vi "toStringArray.vi"(8 "error in (no error)":errorcluster, 11 "SingleTone in":refnum<class "SingleTone.lvclass">) -> (0 "error out":errorcluster, 2 "eventStringArray":string[](array[string]), 3 "SingleTone out":refnum<class "SingleTone.lvclass">)   [LabVIEW 2011, in "Tools.lvlib" / "Scripting.lvlib" / "SingleTone.lvclass"]
uses:
  SingleTone.lvclass
  ScriptEvent.lvclass
  SingleTone.lvclass/SingleTone.ctl
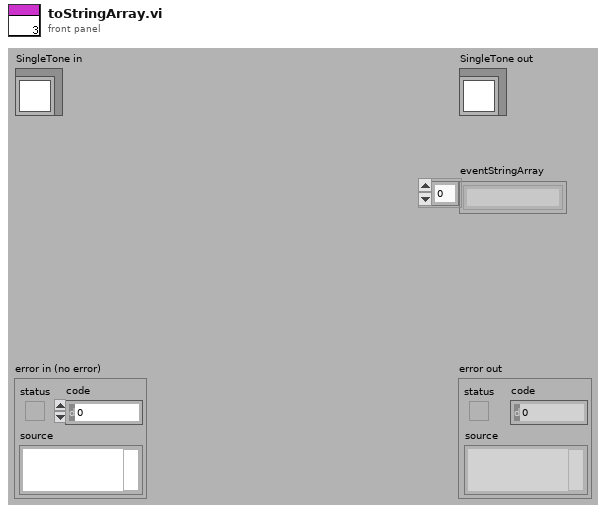
[diagram p1: front panel]
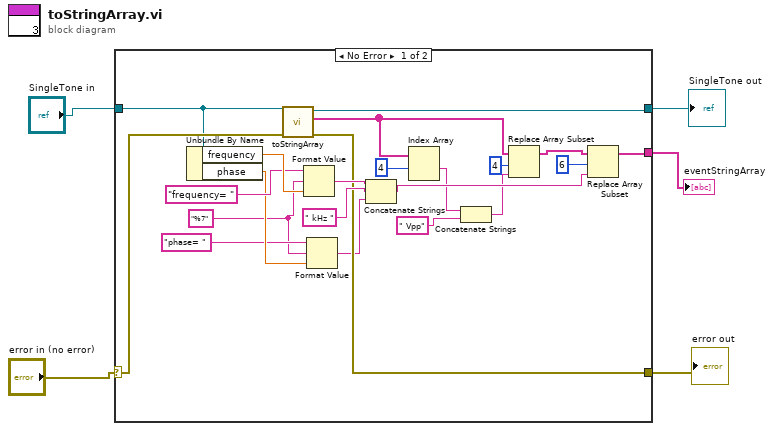
[diagram p0: block diagram]
diagram:
  n1 = case shown="No Error" "error in (no error)" {
    selector: "error in (no error)" -> [w25 w29]
    tunnel: [w17 w29] -> w1
    tunnel: [w27 w28] -> w3
    tunnel: "SingleTone in" -> [w24 w28]
    tunnel: [w18 _] -> w2
    frame No Error {
      w9 = "%7"
      n2 = Unbundle By Name(w24) -> ("frequency"=w23:dbl, "phase"=w11:dbl)
      n3 = call-parent "toStringArray.vi"("error in (no error)"=w25, "ScriptEvent in"=w24) -> ("error out"=w17:errorcluster, "eventStringArray"=w7:string[], "ScriptEvent out"=w27:refnum<class "SingleTone.lvclass">)  [unwired: 7 in]
      n4 = Format Value(string ("")="frequency= ", format string=w9, value (0)=w23) -> (output string=w21:string)
      n5 = Format Value(string ("")="phase= ", format string=w9, value (0)=w11) -> (output string=w8:string)
      n6 = Concatenate Strings(w21, " kHz ", w8) -> (w19:string)
      n7 = Index Array(array=w7, index #1=4) -> (element #1=w14:string)  [unwired: 1 in, 1 out]
      n8 = Concatenate Strings(w14, " Vpp") -> (w12:string)
      n9 = Replace Array Subset(array=w7, new element=w12, index=4) -> (w6:string[])
      n10 = Replace Array Subset(array=w6, new element=w19, index=6) -> (w18:string[])
    }
    frame Error {
    }
  }
  "error out" <- w1
  "SingleTone out" <- w3
  "eventStringArray" <- w2
